vi "NI_PCIE_6509_DO.vi"(11 "Queue Ref In":T1={"UI"=refnum, "Message"=refnum, "Data"=refnum, "Caller"=refnum, "Name"="000 Common", "Data Path"=path "", "Class Path"=path "", "SubPanel"=refnum, "Project Name"="", "MNT"="", "Title"="", "Data Source"=refnum, "Queue List"={}, "VI"=refnum, "UE"=refnum}) -> ()   [LabVIEW 2020]
doc: "PCIE_6509"
uses:
  Alin/QMH/000 Module Data Type.ctl
  Alin/QMH/Queue Message.ctl
  9999 SubVI/Global/Data Global/SDQ Data Type.ctl
  <vilib>/DAQmx/write.llb/DAQmx Write (Digital 1D Bool NChan 1Samp 1Line).vi
  <vilib>/Utility/file.llb/Write Delimited Spreadsheet (string).vi
  <vilib>/DAQmx/create/channels.llb/DAQmx Create Channel (DO-Digital Output).vi
  <vilib>/DAQmx/miscellaneous.llb/DAQmx Fill In Error Info.vi
  <resource>/objmgr/daqmx.rc
panel:
  out "Type":map{string, string}(c390)
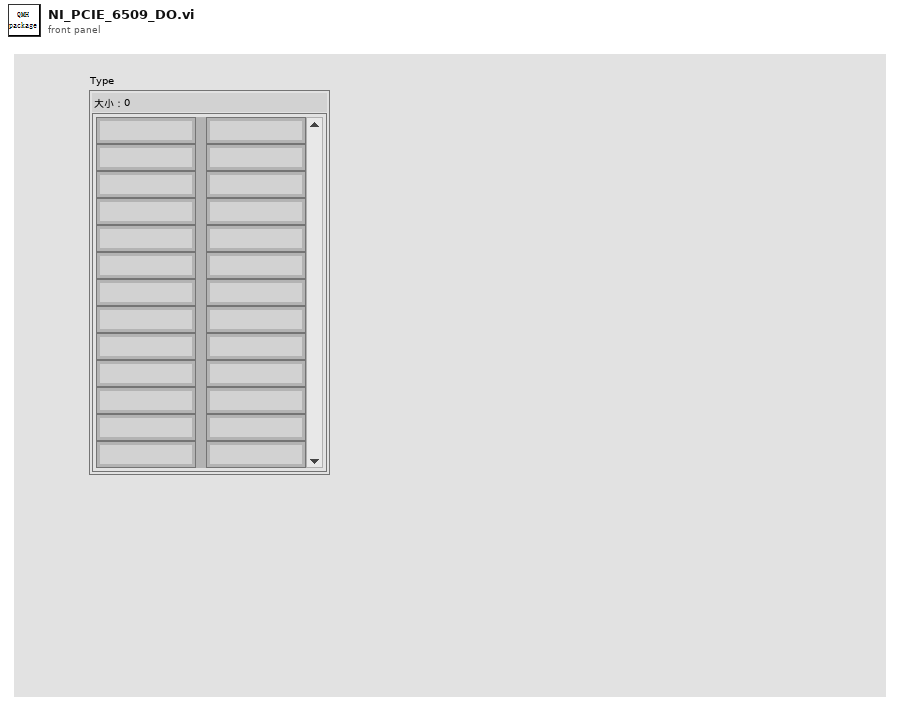
[diagram p1: front panel]
types:
  T1 = typedef "000 Module Data Type.ctl" = cluster{"UI":refnum<queue>, "Message":refnum<queue>, "Data":refnum<queue>, "Caller":refnum<queue>, "Name":string, "Data Path":path, "Class Path":path, "SubPanel":refnum<vi>, "Project Name":string, "MNT":string, "Title":string, "Data Source":refnum<queue>, "Queue List":map{string, refnum<queue>}, "VI":refnum<vi>, "UE":refnum<user-event>}
  T2 = typedef "SDQ Data Type.ctl" = cluster{"CAN Length":string, "CAN Name":string, "CAN ID":string, "CAN Type":string, "Test Item":string, "Byte Order":string, "Instruction":string, "Control Type":string, "Group":string, "Offset":dbl, "Coefficient":dbl, "Write Enable":bool, "Lable Type":string, "Key?":string, "Set Value":string, "Upper":dbl, "Lower":dbl, "Unit":string, "Formula":string, "Test Item Type":string, "Length":i32, "Address":string, "Name":string, "Identifier":string, "Data Type":string, "Enumerate?":string, "Enumerate List":string, "Data":string, "Source":string}
  T3 = cluster{"Queue":T1, "Delay":cluster{"Count Time(ms)":u32, "Delay Time(ms)":u32, "Next":string}, "Data":map{string, T2}, "PCIE_6509":cluster{"Port":string, "Task":refnum<k21>}, "IDS":string[], "Type":map{string, string}, "Title":string[]}
  T4 = typedef "005 Data Source Type.ctl" = cluster{"Device Name":string, "Device Model":string, "Device Driver":string, "IP Address":string, "Port":string, "Remark":string, "Enable":string, "Path":string}
  T5 = cluster{"Name":string, "Type":map{string, string}}
  T6 = typedef "eventvkey.ctl" = enum16{"ASCII", "Enter", "Return", "Shift", "Ctrl", "Alt", "Cmd", "Opt", "Caps", "NumLock", "Clear", "Break", "Up", "Down", "Left", "Right", "Insert", "Delete", "Home", "End", "PageUp", "PageDown", "Escape", "Help", "Pause", "ScrollLock", "F1", "F2", "F3", "F4", "F5", "F6", "F7", "F8", "F9", "F10", "F11", "F12", "F13", "F14", "F15", "F16", "F17", "F18", "F19", "F20", "F21", "F22", "F23", "F24", "Play", "VolumeUp", "VolumeDown", "Mute", "Two Byte Char"}
  T7 = cluster{"Shift":bool, "Ctrl":bool, "Alt":bool, "Cmd":bool, "Opt":bool}
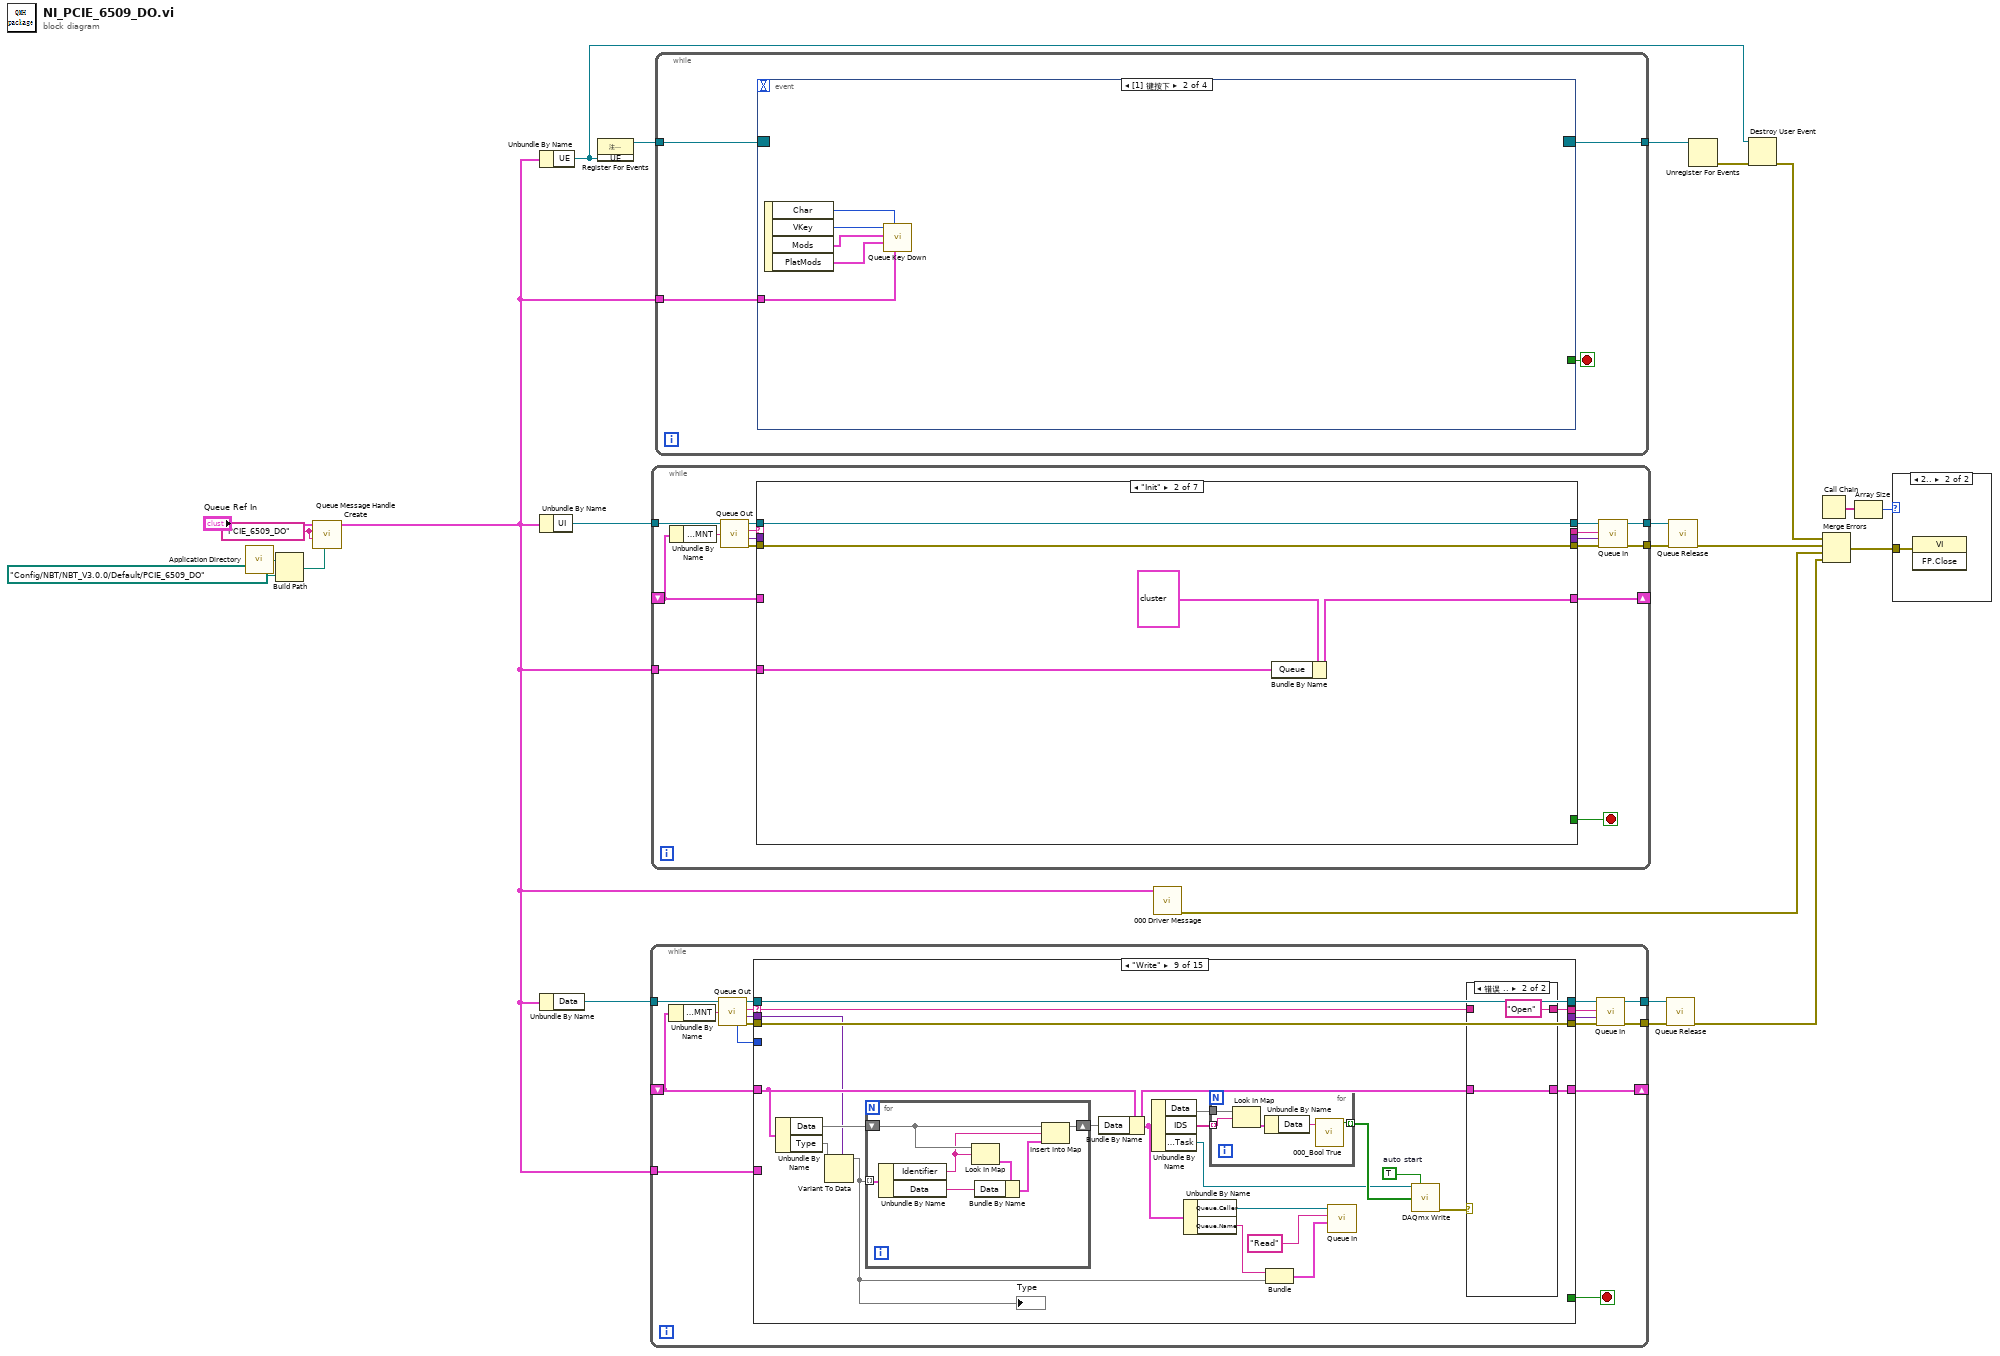
[diagram p0: block diagram]
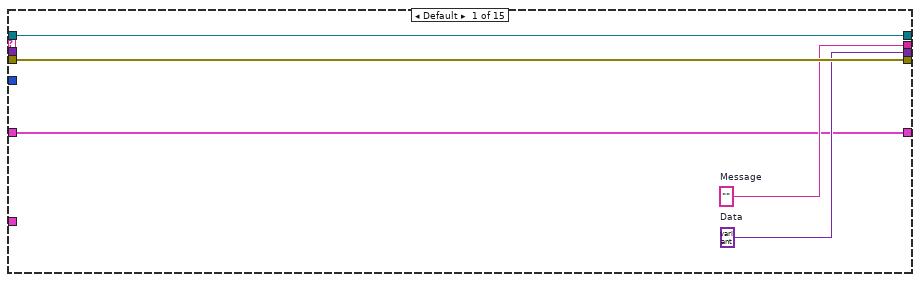
[diagram p2: hidden frame]
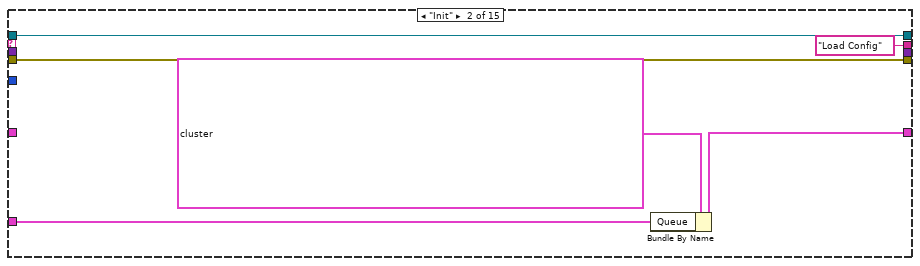
[diagram p3: hidden frame]
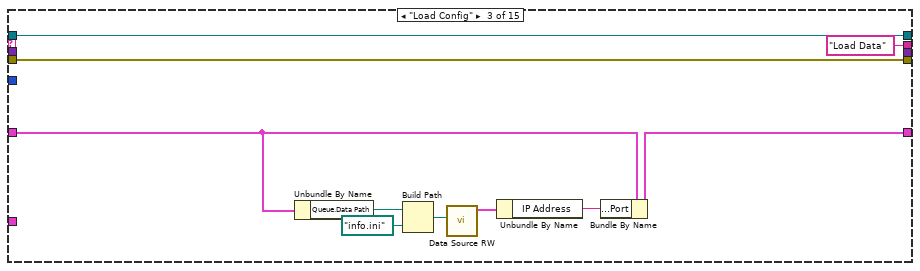
[diagram p4: hidden frame]
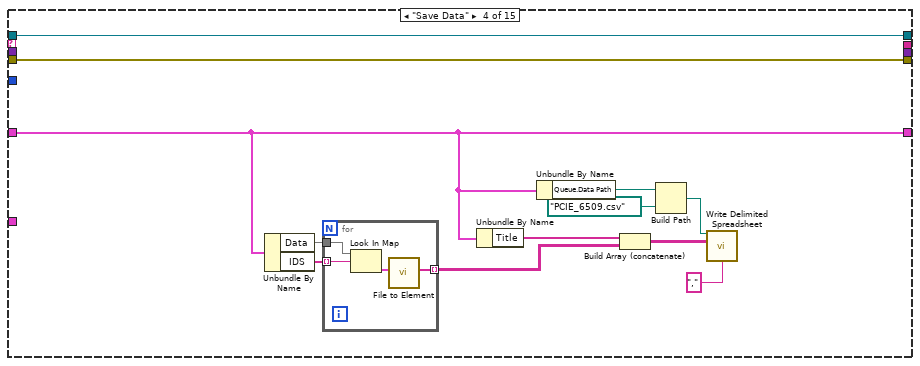
[diagram p5: hidden frame]
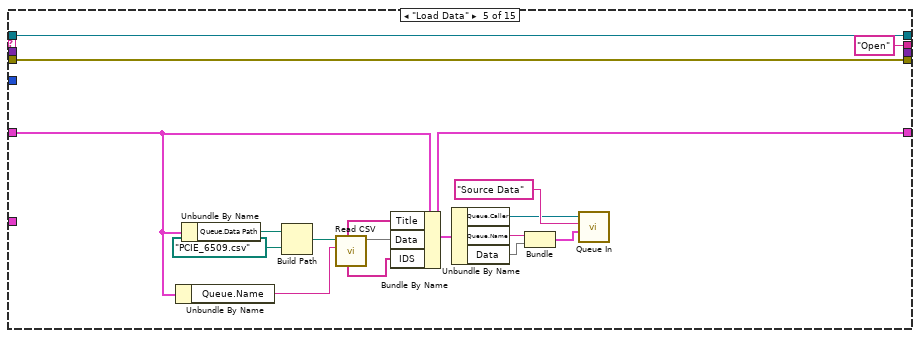
[diagram p6: hidden frame]
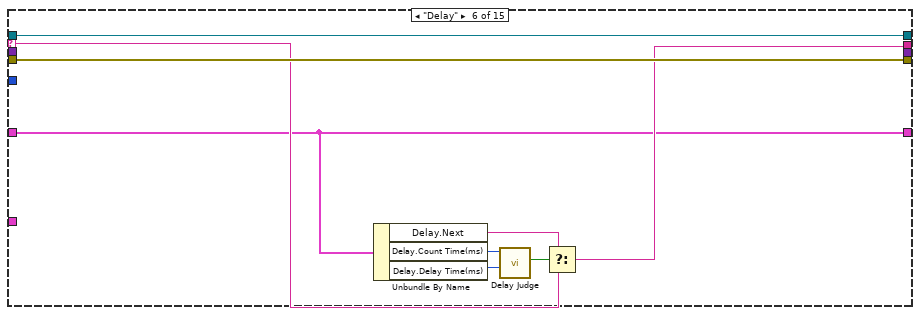
[diagram p7: hidden frame]
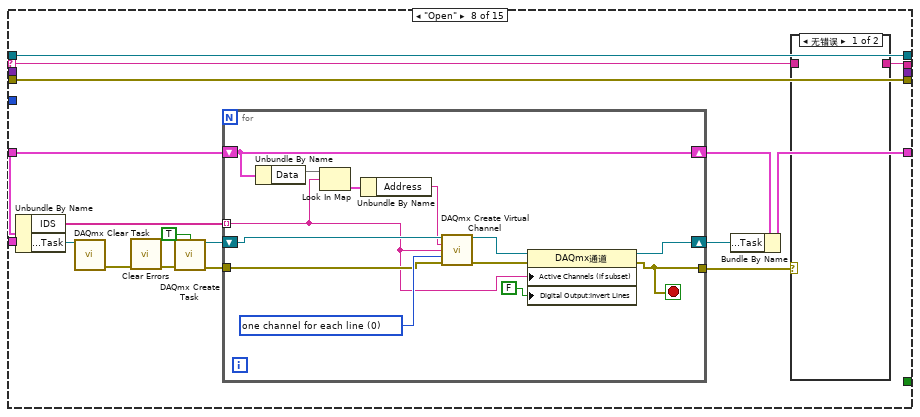
[diagram p9: hidden frame]
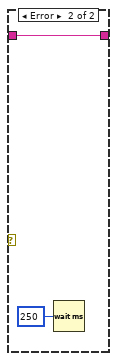
[diagram p10: hidden frame]
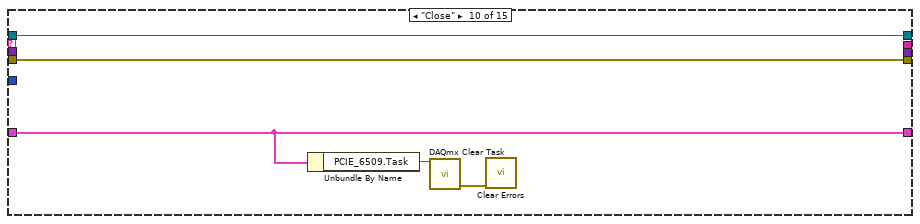
[diagram p12: hidden frame]
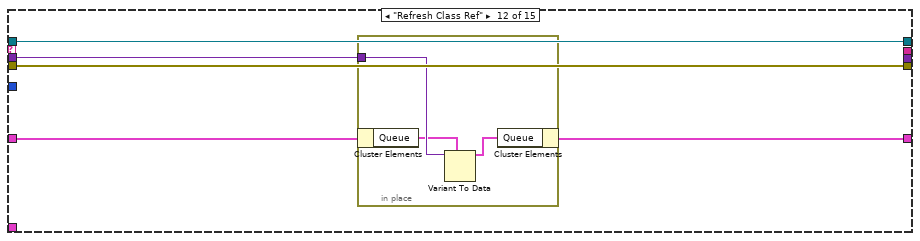
[diagram p14: hidden frame]
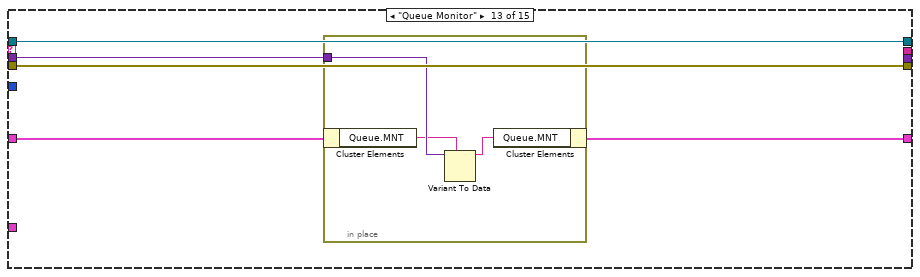
[diagram p15: hidden frame]
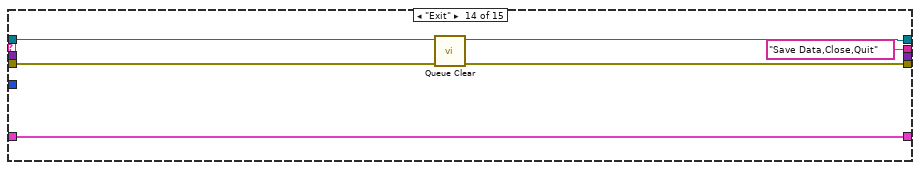
[diagram p16: hidden frame]
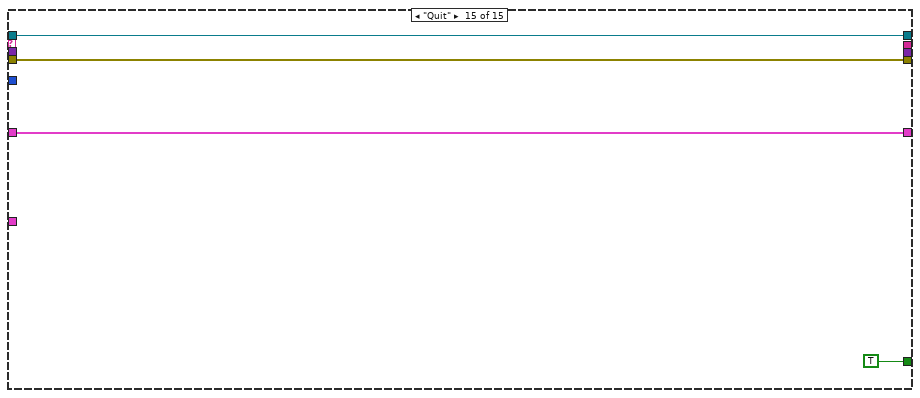
[diagram p17: hidden frame]
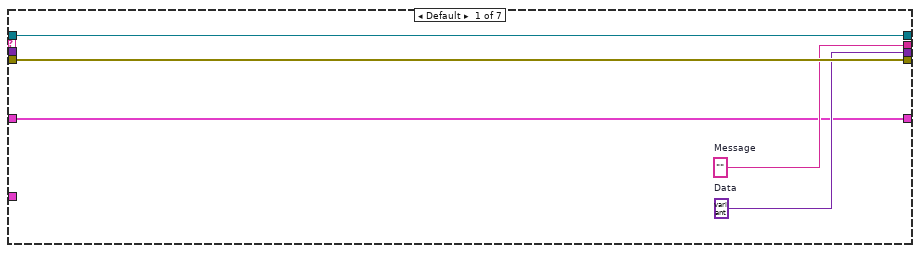
[diagram p19: hidden frame]
diagram:
  w1 = "PCIE_6509_DO" ("Title")
  n1 = call <vilib>:"Application Directory.vi"() -> ("Application Directory"=w4:path)
  n2 = Build Path(base path=w4, name or relative path=path "Config/NBT/NBT_V3.0.0/Default/PCIE_6509_DO" ("名称或相对路径")) -> (appended path=w2:path)
  n3 = call "Queue Message Handle Create.vi"("Data Path"=w2, "Name"=w1, "Title"=w1, "Queue Ref In"="Queue Ref In") -> ("Queue Ref Out"=w5:T1)  [unwired: 6 in, 1 out]
  n4 = Unbundle By Name(w5) -> ("UE"=w7:refnum<user-event>)
  n5 = Unbundle By Name(w5) -> ("UI"=w18:refnum<queue>)
  n6 = Unbundle By Name(w5) -> ("Data"=w10:refnum<queue>)
  n7 = register-events(w7) -> (reference out=w23:refnum<event-registration>)  [unwired: 2 in, 1 out]
  n8 = while {
    tunnel: w10 -> [w36]
    tunnel: [w33] -> w12
    tunnel: [w32] -> w11
    shift-right: [w28] -> _
    shift-left: _ -> [w25]
    tunnel: w5 -> [w24]
    stop <- w40 stop-if-true
    n9 = Unbundle By Name(w25) -> ("Queue.MNT"=w26:string)
    n10 = call "Queue Out.vi"("Monitor"=w26, "Queue In"=w36) -> ("error out"=w39:errorcluster, "Data"=w37:variant, "Message"=w38:string, "Queue Out"=w35:refnum<queue>, "Queue NUmber"=w27:i32)  [unwired: 5 in]
    n11 = case shown="\"Write\"" w38 {
      selector: w38 -> [_ _ _ _ _ w96 _ w112 w154 _ _ _ _ _ _]
      tunnel: w35 -> [w45 w51 w61 w73 w94 w103 w106 w122 w159 w179 w182 w187 w195 w203 w207]
      tunnel: w39 -> [w44 w50 w60 w72 w93 w102 w105 w121 w158 w178 w181 w186 w194 w201 w208]
      tunnel: [w45 w51 w61 w73 w94 w103 w106 w122 w159 w179 w182 w187 w195 w202 w207] -> w34
      tunnel: [w44 w50 w60 w72 w93 w102 w105 w121 w158 w178 w181 w186 w194 w200 w208] -> w31
      tunnel: [w43 "Load Config" ("Next") "Load Data" ("Next") _ "Open" ("Next") w97 _ w111 w153 _ _ _ _ "Save Data,Close,Quit" _] -> w30
      tunnel: [_ _ _ _ _ _ _ _ _ _ _ _ _ _ TRUE] -> w40
      tunnel: [w42 _ _ _ _ _ _ _ _ _ _ _ _ _ _] -> w29
      tunnel: w37 -> [_ _ _ _ _ _ _ _ w145 _ _ w183 w191 _ _]
      tunnel: [w41 w47 w53 w64 w83 w95 w104 w119 w155 w177 w180 w184 w192 w199 w205] -> w28
      tunnel: w25 -> [w41 _ w58 w64 w79 w95 w104 w109 w156 w177 w180 w185 w193 w199 w205]
      tunnel: w27 -> [_ _ _ _ _ _ _ _ _ _ _ _ _ _ _]
      tunnel: w24 -> [_ w46 _ _ _ _ _ _ _ _ _ _ _ _ _]
      frame Default {
        w42 = variant  # Data
        w43 = ""  # Message
      }
      frame "Init" {
        n12 = Bundle By Name(cluster=T3 {"Queue"={"UI"=refnum, "Message"=refnum, "Data"=refnum, "Caller"=refnum, "Name"="000 Common", "Data Path"=path "", "Class Path"=path "", "SubPanel"=refnum, "Project Name"="", "MNT"="", "Title"="", "Data Source"=refnum, "Queue List"={}, "VI"=refnum, "UE"=refnum}, "Delay"={"Count Time(ms)"=250, "Delay Time(ms)"=250, "Next"="Receive Data,Delay"}, "Data"={}, "PCIE_6509"={"Port"="", "Task"=""}, "IDS"=[], "Type"={}, "Title"=[]}, "Queue"=w46) -> (w47:T3)
      }
      frame "Load Config" {
        n13 = Unbundle By Name(w58) -> ("Queue.Data Path"=w57:path)
        n14 = Build Path(base path=w57, name or relative path=path "info.ini" ("名称或相对路径")) -> (appended path=w55:path)
        n15 = call "Data Source RW.vi"("Source Path"=w55) -> ("Data Type Out"=w54:T4)  [unwired: 7 in, 3 out]
        n16 = Unbundle By Name(w54) -> ("IP Address"=w52:string)
        n17 = Bundle By Name(cluster=w58, "PCIE_6509.Port"=w52) -> (w53:T3)
      }
      frame "Save Data" {
        n18 = Unbundle By Name(w64) -> ("Data"=w62:map{string, T2}, "IDS"=w70:string[])
        n19 = for {
          tunnel: w70 -> [w75] mode=indexing
          tunnel: [w76] -> w68 mode=indexing
          tunnel: w62 -> [w74]
          n20 = Look In Map(map=w74, key=w75) -> (value=w77:T2)  [unwired: 1 in, 1 out]
          n21 = call "File to Element.vi"("Element In"=w77) -> ("Data Out"=w76:string[])  [unwired: 9 in, 1 out]
        }
        n22 = Unbundle By Name(w64) -> ("Title"=w69:string[])
        n23 = Unbundle By Name(w64) -> ("Queue.Data Path"=w63:path)
        n24 = Build Array (concatenate)(w69, w68) -> (w67:string[][])
        n25 = Build Path(base path=w63, name or relative path=path "PCIE_6509.csv" ("名称或相对路径")) -> (appended path=w65:path)
        n26 = call-poly <vilib>:"Write Delimited Spreadsheet.vi"("file path (dialog if empty)"=w65, "2D data"=w67, "delimiter (\\t)"="," ("delimiter (\\t)")) -> ()  [unwired: 11 in, 2 out]
      }
      frame "Load Data" {
        n27 = Unbundle By Name(w79) -> ("Queue.Name"=w78:string)
        n28 = Unbundle By Name(w79) -> ("Queue.Data Path"=w92:path)
        n29 = Build Path(base path=w92, name or relative path=path "PCIE_6509.csv" ("名称或相对路径")) -> (appended path=w90:path)
        n30 = call "Read CSV.vi"("Source"=w78, "Data Path"=w90) -> (3:"Identifiers Out"=w89:map{string, T2}, 6:"Identifiers Out"=w82:string[], "Title"=w80:string[])  [unwired: 2 in, 5 out]
        n31 = Bundle By Name(cluster=w79, "Title"=w80, "Data"=w89, "IDS"=w82) -> (w83:T3)
        n32 = Unbundle By Name(w83) -> ("Queue.Caller"=w84:refnum<queue>, "Queue.Name"=w88:string, "Data"=w86:map{string, T2})
        n33 = Bundle("Name"=w88, "Data"=w86) -> (w87:cluster{"Name":string, "Data":map{string, T2}})  [unwired: 1 in]
        n34 = call "Queue In.vi"("Data"=w87, "Message"="Source Data", "Queue In"=w84) -> ()  [unwired: 7 in, 2 out]
      }
      frame "Delay" {
        n35 = Unbundle By Name(w95) -> ("Delay.Next"=w101:string, "Delay.Count Time(ms)"=w98:u32, "Delay.Delay Time(ms)"=w99:u32)
        n36 = call "Delay Judge.vi"("Delay Time(ms)"=w99, "Count Time(ms)"=w98) -> ("Time Out?"=w100:bool)  [unwired: 5 in, 4 out]
        n37 = Select(t=w101, s=w100, f=w96) -> (s? t:f=w97:string)
      }
      frame "===Driver====" {
      }
      frame "Open" {
        n38 = Unbundle By Name(w109) -> ("IDS"=w110:string[], "PCIE_6509.Task"=w118:refnum<k21>)
        n39 = call <vilib>:"DAQmx Clear Task.vi"("task in"=w118) -> ("error out"=w117:errorcluster)  [unwired: 14 in]
        n40 = call <vilib>:"Clear Errors.vi"("error in (no error)"=w117) -> ("error out"=w116:errorcluster)  [unwired: 5 in, 1 out]
        n41 = call <vilib>:"DAQmx Create Task.vi"("auto cleanup"=TRUE, "error in"=w116) -> ("task out"=w115:refnum<k21>, "error out"=w107:errorcluster)  [unwired: 12 in]
        n42 = for {
          shift-right: [w130] -> w114
          shift-left: w115 -> [w128]
          tunnel: [w125] -> w113
          tunnel: w110 -> [w126] mode=indexing
          shift-right: [w137] -> w108
          shift-left: w109 -> [w137]
          tunnel: w107 -> [w129]
          stop <- w125 stop-if-true
          w132 = 0 items=["one channel for each line", "one channel for all lines"] ("line grouping")
          n43 = Unbundle By Name(w137) -> ("Data"=w136:map{string, T2})
          n44 = Look In Map(map=w136, key=w126) -> (value=w135:T2)  [unwired: 1 in, 1 out]
          n45 = Unbundle By Name(w135) -> ("Address"=w127:string)
          n46 = call-poly <vilib>:"DAQmx Create Virtual Channel.vi"("task in"=w128, "lines"=w127, "name to assign"=w126, "line grouping"=w132, "error in"=w129) -> ("task out"=w134:refnum<k21>, "error out"=w133:errorcluster)  [unwired: 9 in]
          n47 = property class="DAQmx通道"(reference=w134, error in=w133, "Active Channels (if subset)"=w126, "Digital Output:Invert Lines"=FALSE ("invert line")) -> (reference out=w130:refnum<k21>, error out=w125:errorcluster)
        }
        n48 = Bundle By Name(cluster=w108, "PCIE_6509.Task"=w114) -> (w119:T3)
        n49 = case shown="无错误" w113 {
          tunnel: w112 -> [_ w124]
          tunnel: [_ w124] -> w111
          frame No Error {
          }
          frame Error {
            n50 = Wait (ms)(milliseconds to wait=u32 250 ("等待时间（毫秒）")) -> ()  [unwired: 1 out]
          }
        }
      }
      frame "Write" {
        w152 = TRUE  # auto start
        n51 = Unbundle By Name(w156) -> ("Data"=w157:map{string, T2}, "Type"=w144:map{string, string})
        n52 = Variant To Data(type=w144, Variant=w145) -> (data=w138:map{string, string})  [unwired: 1 in, 1 out]
        "Type" <- w138
        n53 = for {
          tunnel: w138 -> [w174] mode=indexing
          shift-right: [w171] -> w151
          shift-left: w157 -> [w172]
          n54 = Unbundle By Name(w174) -> ("Identifier"=w169:string, "Data"=w168:string)
          n55 = Look In Map(map=w172, key=w169) -> (value=w173:T2)  [unwired: 1 in, 1 out]
          n56 = Bundle By Name(cluster=w173, "Data"=w168) -> (w170:T2)
          n57 = Insert Into Map(map in=w172, key=w169, value=w170) -> (map out=w171:map{string, T2})  [unwired: 2 out]
        }
        n58 = Bundle By Name(cluster=w156, "Data"=w151) -> (w141:T3)
        n59 = Unbundle By Name(w141) -> ("Data"=w148:map{string, T2}, "IDS"=w149:string[], "PCIE_6509.Task"=w146:refnum<k21>)
        n60 = Unbundle By Name(w141) -> ("Queue.Caller"=w140:refnum<queue>, "Queue.Name"=w139:string)
        n61 = for {
          tunnel: w149 -> [w163] mode=indexing
          tunnel: w148 -> [w164]
          tunnel: [w160] -> w147 mode=indexing
          n62 = Look In Map(map=w164, key=w163) -> (value=w162:T2)  [unwired: 1 in, 1 out]
          n63 = Unbundle By Name(w162) -> ("Data"=w161:string)
          n64 = call "000_Bool True.vi"("Bool String"=w161) -> ("True"=w160:bool)  [unwired: 8 in, 2 out]
        }
        n65 = Bundle("Name"=w139, "Type"=w138) -> (w143:T5)  [unwired: 1 in]
        n66 = call "Queue In.vi"("Data"=w143, "Message"="Read", "Queue In"=w140) -> ()  [unwired: 7 in, 2 out]
        n67 = call-poly <vilib>:"DAQmx Write.vi"("task/channels in"=w146, "auto start"=w152, "data"=w147) -> ("error out"=w150:errorcluster)  [unwired: 10 in, 2 out]
        n68 = case shown="错误 .." w150 {
          tunnel: w141 -> [w165 w167]
          tunnel: [w165 w167] -> w155
          tunnel: w154 -> [_ _]
          tunnel: [_ "Open"] -> w153
          frame No Error {
          }
          frame Error {
          }
        }
      }
      frame "Close" {
        n69 = Unbundle By Name(w177) -> ("PCIE_6509.Task"=w176:refnum<k21>)
        n70 = call <vilib>:"DAQmx Clear Task.vi"("task in"=w176) -> ("error out"=w175:errorcluster)  [unwired: 14 in]
        n71 = call <vilib>:"Clear Errors.vi"("error in (no error)"=w175) -> ()  [unwired: 5 in, 2 out]
      }
      frame "====System====" {
      }
      frame "Refresh Class Ref" {
        n72 = in-place {
          in-place-border: w183 -> [w190]
          n73 = in-place-cluster #1(w185) -> ("Queue"=w189:T1)
          n74 = Variant To Data(type=w189, Variant=w190) -> (data=w188:T1)  [unwired: 1 in, 1 out]
          n75 = in-place-cluster #1("Queue"=w188) -> (w184:T3)
        }
      }
      frame "Queue Monitor" {
        n76 = in-place {
          in-place-border: w191 -> [w198]
          n77 = in-place-cluster #2(w193) -> ("Queue.MNT"=w197:string)
          n78 = Variant To Data(type=w197, Variant=w198) -> (data=w196:string)  [unwired: 1 in, 1 out]
          n79 = in-place-cluster #2("Queue.MNT"=w196) -> (w192:T3)
        }
      }
      frame "Exit" {
        n80 = call "Queue Clear.vi"("error in (no error)"=w201, "Queue In"=w203) -> ("error out"=w200:errorcluster, "Queue Out"=w202:refnum<queue>)  [unwired: 8 in]
      }
      frame "Quit" {
      }
    }
    n81 = call "Queue In.vi"("error in (no error)"=w31, "Data"=w29, "Message"=w30, "Queue In"=w34) -> ("error out"=w32:errorcluster, "Queue Out"=w33:refnum<queue>)  [unwired: 6 in]
  }
  n82 = while {
    tunnel: w18 -> [w220]
    tunnel: [w217] -> w20
    tunnel: [w216] -> w19
    shift-right: [w212] -> _
    shift-left: _ -> [w211]
    tunnel: w5 -> [w209]
    stop <- w224 stop-if-true
    n83 = Unbundle By Name(w211) -> ("Queue.MNT"=w210:string)
    n84 = call "Queue Out.vi"("Monitor"=w210, "Queue In"=w220) -> ("error out"=w223:errorcluster, "Data"=w221:variant, "Message"=w222:string, "Queue Out"=w219:refnum<queue>)  [unwired: 5 in, 1 out]
    n85 = case shown="\"Init\"" w222 {
      selector: w222 -> [_ _ _ _ _ w256 _]
      tunnel: w219 -> [w229 w234 w237 w242 w250 w263 w269]
      tunnel: w223 -> [w228 w233 w236 w241 w249 w261 w270]
      tunnel: [w229 w234 w237 w242 w250 w262 w269] -> w218
      tunnel: [w228 w233 w236 w241 w249 w260 w270] -> w215
      tunnel: [w227 _ _ _ _ "Quit" _] -> w214
      tunnel: [_ _ _ _ _ _ TRUE] -> w224
      tunnel: [w226 _ _ _ _ _ _] -> w213
      tunnel: w221 -> [_ _ _ w238 w246 _ _]
      tunnel: [w225 w231 w235 w239 w247 w255 w267] -> w212
      tunnel: w211 -> [w225 _ w235 w240 w248 w255 w267]
      tunnel: w209 -> [_ w230 _ _ _ _ _]
      frame Default {
        w226 = variant  # Data
        w227 = ""  # Message
      }
      frame "Init" {
        n86 = Bundle By Name(cluster=cluster{"Queue":T1} {"Queue"={"UI"=refnum, "Message"=refnum, "Data"=refnum, "Caller"=refnum, "Name"="000 Common", "Data Path"=path "", "Class Path"=path "", "SubPanel"=refnum, "Project Name"="", "MNT"="", "Title"="", "Data Source"=refnum, "Queue List"={}, "VI"=refnum, "UE"=refnum}}, "Queue"=w230) -> (w231:cluster{"Queue":T1})
      }
      frame "====System====" {
      }
      frame "Refresh Class Ref" {
        n87 = in-place {
          in-place-border: w238 -> [w245]
          n88 = in-place-cluster #3(w240) -> ("Queue"=w244:T1)
          n89 = Variant To Data(type=w244, Variant=w245) -> (data=w243:T1)  [unwired: 1 in, 1 out]
          n90 = in-place-cluster #3("Queue"=w243) -> (w239:cluster{"Queue":T1})
        }
      }
      frame "Queue Monitor" {
        n91 = in-place {
          in-place-border: w246 -> [w253]
          n92 = in-place-cluster #4(w248) -> ("Queue.MNT"=w252:string)
          n93 = Variant To Data(type=w252, Variant=w253) -> (data=w251:string)  [unwired: 1 in, 1 out]
          n94 = in-place-cluster #4("Queue.MNT"=w251) -> (w247:cluster{"Queue":T1})
        }
      }
      frame "Exit" {
        n95 = Unbundle By Name(w255) -> ("Queue.Message"=w259:refnum<queue>, "Queue.Data"=w258:refnum<queue>, "Queue.UE"=w254:refnum<user-event>)
        n96 = Build Array(w259, w258) -> (w257:refnum<queue>[])
        n97 = Generate User Event(user event=w254, event data cluster=w256) -> ()  [unwired: 2 in, 2 out]
        n98 = for {
          tunnel: w257 -> [w266] mode=indexing
          tunnel: w256 -> [w265]
          n99 = call "Queue In.vi"("Message"=w265, "Queue In"=w266) -> ()  [unwired: 8 in, 2 out]
        }
        n100 = call "Queue Clear.vi"("error in (no error)"=w261, "Queue In"=w263) -> ("error out"=w260:errorcluster, "Queue Out"=w262:refnum<queue>)  [unwired: 8 in]
      }
      frame "Quit" {
      }
    }
    n101 = call "Queue In.vi"("error in (no error)"=w215, "Data"=w213, "Message"=w214, "Queue In"=w218) -> ("error out"=w216:errorcluster, "Queue Out"=w217:refnum<queue>)  [unwired: 6 in]
  }
  n102 = while {
    tunnel: w23 -> [w274]
    tunnel: [w272] -> w22
    tunnel: w5 -> [w271]
    stop <- w273 stop-if-true
    n103 = event shown="[1] 键按下" {
      selector: w274 -> [_ _ _ _]
      dyn-events: [_ _ _ _] -> w272
      timeout: _ -> [_ _ _ _]
      tunnel: [_ _ w280 _] -> w273
      tunnel: w271 -> [_ w275 _ w285]
      event Timeout {
        n104 = event-data() -> ()  [unwired: 1 in, 1 out]
      }
      event Key Down {
        n105 = event-data() -> ("Char"=w279:i16, "VKey"=w278:T6, "Mods"=w277:cluster{"Num Pad":bool, "Menu Key":bool}, "PlatMods"=w276:T7)  [unwired: 1 in]
        n106 = call "Queue Key Down.vi"("Queue Ref Out"=w275, "C"=w279, "Platform Key"=w276, "Group Key"=w277, "V Key"=w278) -> ()  [unwired: 6 in, 1 out]
      }
      event User Event {
        n107 = event-data() -> ("Message"=w282:string)  [unwired: 1 in]
        n108 = Equal?(x=w282, y="Exit") -> (x = y?=w280:bool)
      }
      event Panel Close? {
        n109 = event-data() -> ()  [unwired: 1 in, 1 out]
        n110 = Call Chain() -> (call chain=w287:string[])
        n111 = Array Size(array=w287) -> (size(s)=w286:i32)
        n112 = case shown="2, 默认" w286 {
          tunnel: w285 -> [w291 w294]
          tunnel: [w290 w293] -> w284
          tunnel: ["Panel Hidden" ("Message") "Exit Prepare" ("Message")] -> w283
          frame 2, Default {
            n113 = Unbundle By Name(w291) -> ("Message"=w290:refnum<queue>)
          }
          frame 1 {
            n114 = Unbundle By Name(w294) -> ("Message"=w293:refnum<queue>)
          }
        }
        n115 = call "Queue In.vi"("Message"=w283, "Queue In"=w284) -> ()  [unwired: 8 in, 2 out]
        n116 = event-data("Discard?"=TRUE ("放弃？")) -> ()  [unwired: 1 in, 1 out]
      }
    }
  }
  n117 = call "000 Driver Message.vi"("Queue In"=w5) -> ("error out"=w8:errorcluster)  [unwired: 8 in, 2 out]
  n118 = call "Queue Release.vi"("error in (no error)"=w11, "Queue In"=w12) -> ("error out"=w9:errorcluster)  [unwired: 9 in]
  n119 = call "Queue Release.vi"("error in (no error)"=w19, "Queue In"=w20) -> ("error out"=w16:errorcluster)  [unwired: 9 in]
  n120 = Unregister For Events(event registration refnum=w22) -> (error out=w21:errorcluster)  [unwired: 1 in]
  n121 = Destroy User Event(user event=w7, error in=w21) -> (error out=w17:errorcluster)
  n122 = Call Chain() -> (call chain=w14:string[])
  n123 = Merge Errors(w17, w16, w8, w9) -> (w15:errorcluster)
  n124 = Array Size(array=w14) -> (size(s)=w13:i32)
  n125 = case shown="2.." w13 {
    tunnel: w15 -> [_ w295]
    frame 0, Default {
    }
    frame 2.. {
      n126 = invoke class="VI" method="FP.Close"(error in=w295) -> ()  [unwired: 2 in, 3 out]
    }
  }
